vi "数据查询_仪器数据.vi"() -> ()   [LabVIEW 2016]
uses:
  <vilib>/Utility/miscctls.llb/LVRowAndColumnUnsignedTypeDef.ctl
  <vilib>/Utility/miscctls.llb/LVPointTypeDef.ctl
  <userlib>/_OpenG.lib/array/array.llb/Sort 2D Array (String)__ogtk.vi
panel:
  in  "序列号":string
  out "总共行数":i32
  in  "显示行数":i32=15
  in  "下拉列表":string(xcontrol)
  in  "导出":bool
  out "分钟小时":string(combo)="实时数据"
  out "工作类型":string(combo)="全部数据"
  in  "查询":bool
  in  "结束日期":string="2050/01/01"
  in  "起始日期":string="2010/01/01"
  out "数据表":string[][](table)
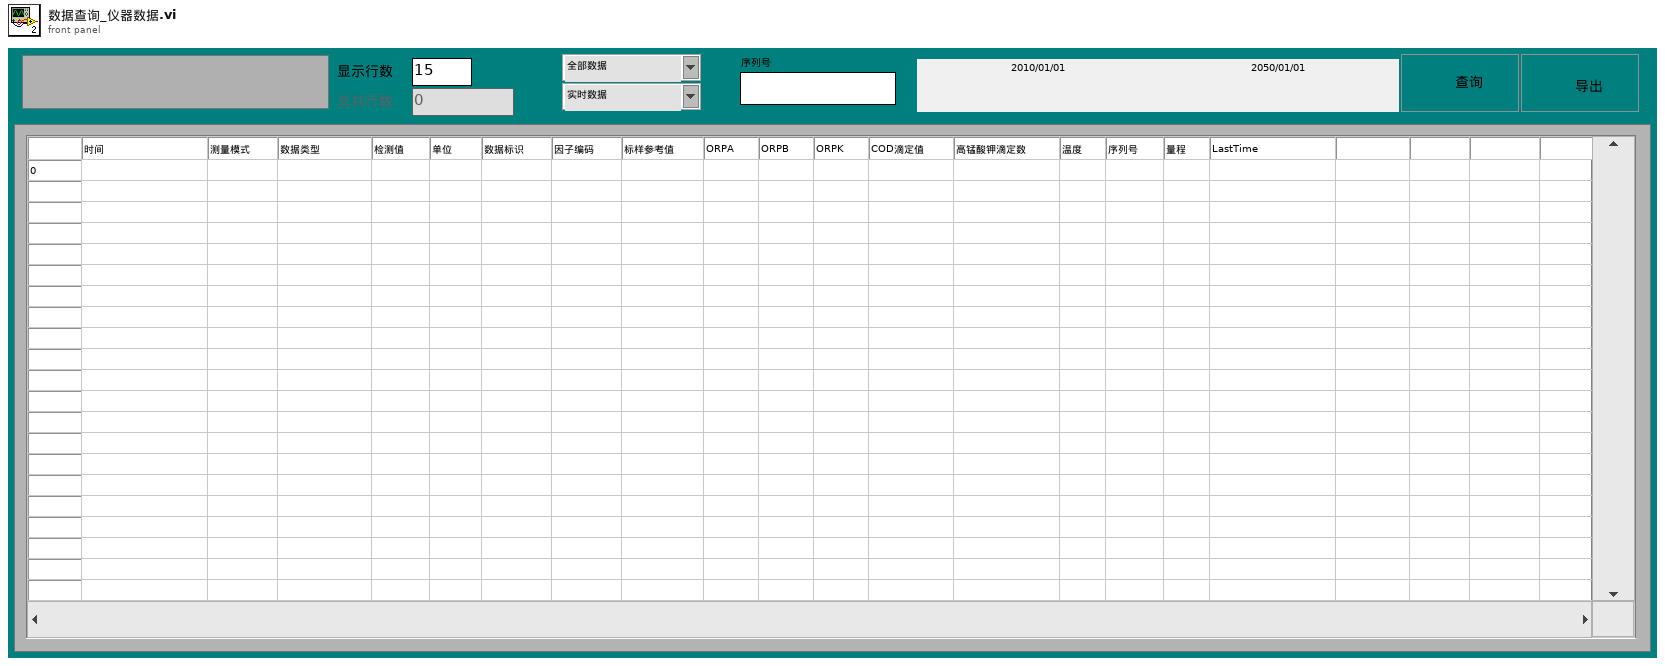
[diagram p1: front panel]
types:
  T1 = enum8{"Enabled", "Disabled", "Disabled and Grayed Out"}
  T2 = typedef "LVRowAndColumnUnsignedTypeDef.ctl" = cluster{"Row":u32, "Column":u32}
  T3 = typedef "LVPointTypeDef.ctl" = cluster{"Horizontal":i16, "Vertical":i16}
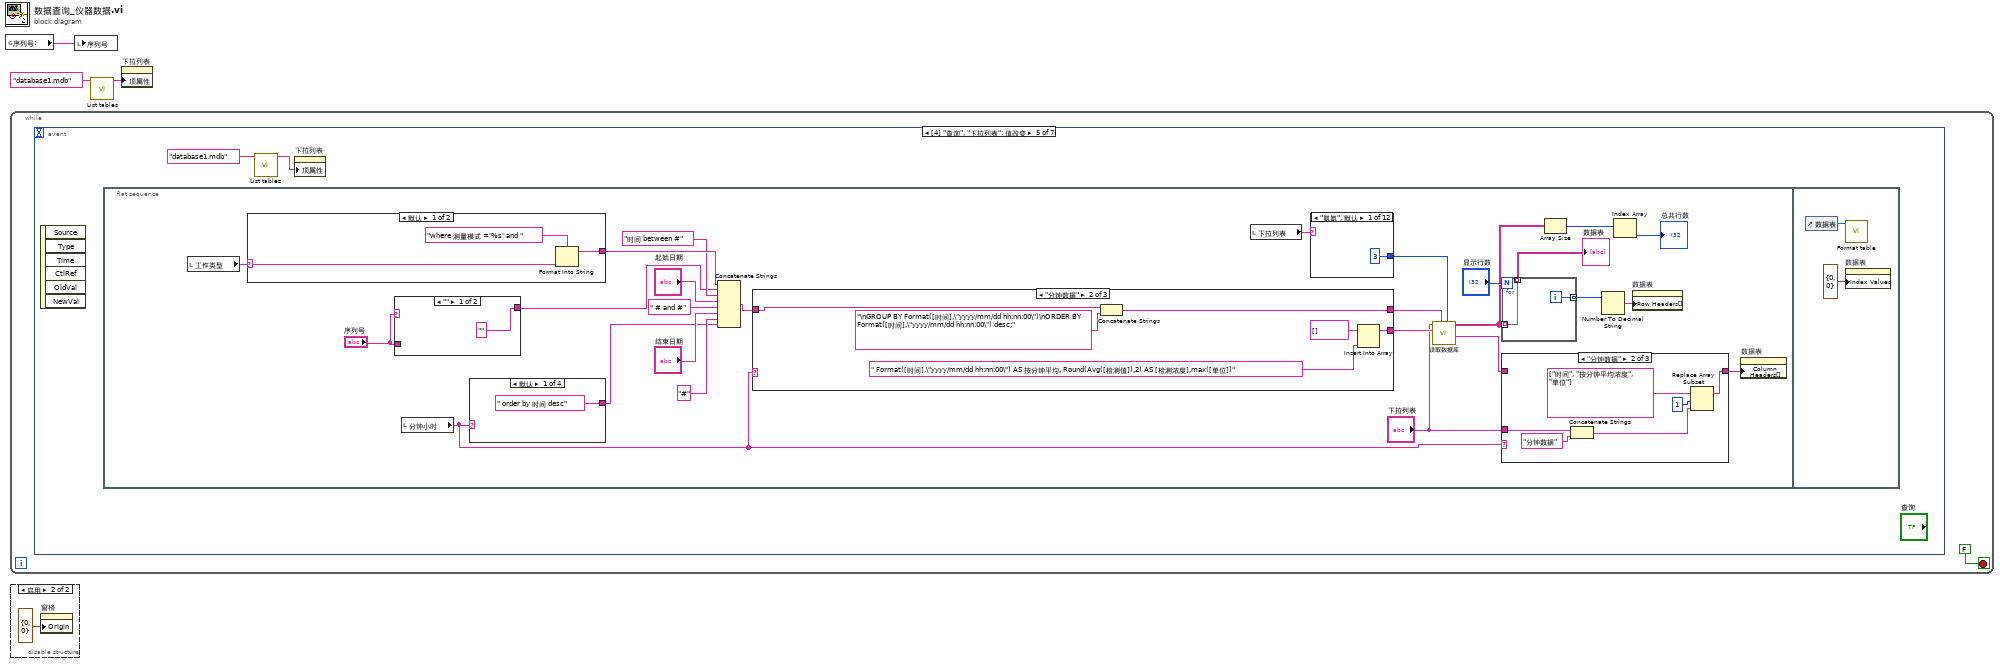
[diagram p0: block diagram]
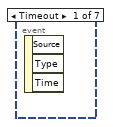
[diagram p2: hidden frame]
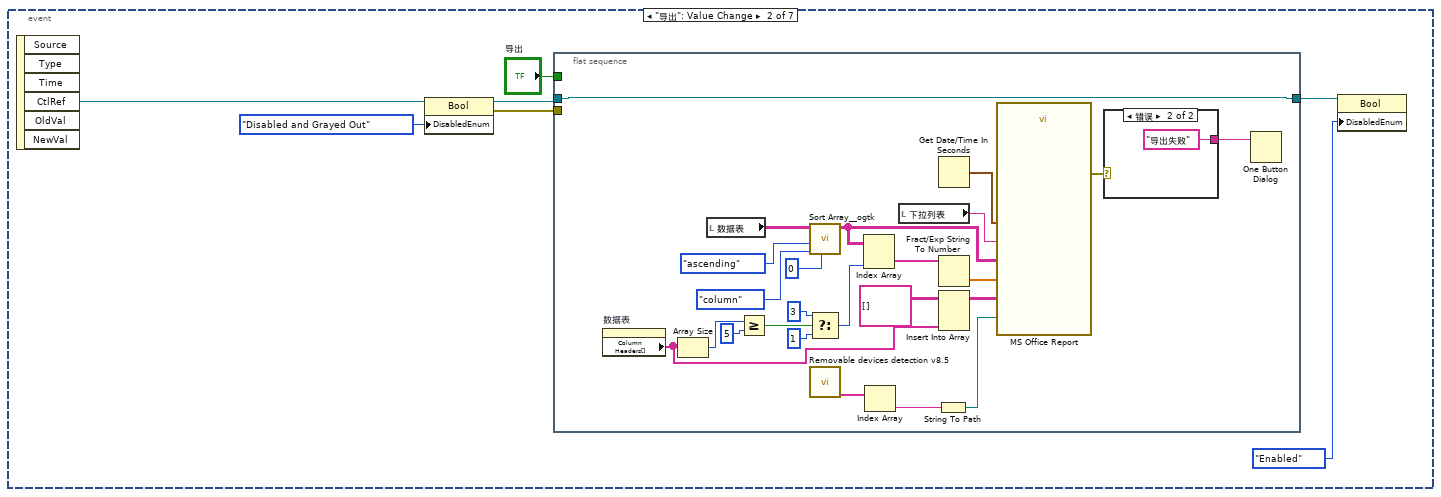
[diagram p3: hidden frame]
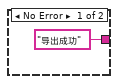
[diagram p4: hidden frame]
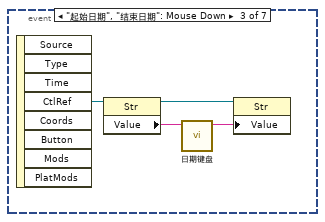
[diagram p5: hidden frame]
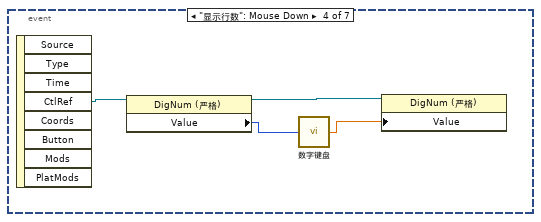
[diagram p6: hidden frame]
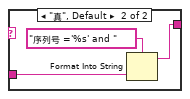
[diagram p7: hidden frame]
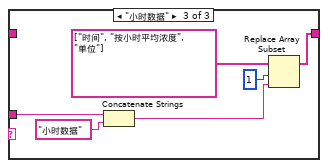
[diagram p9: hidden frame]
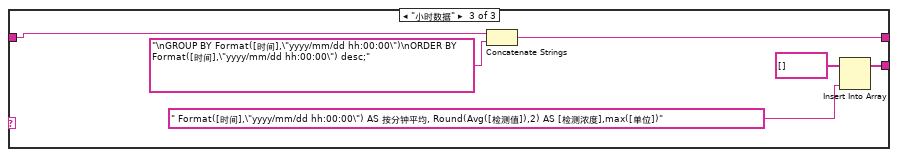
[diagram p14: hidden frame]
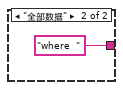
[diagram p15: hidden frame]
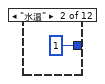
[diagram p16: hidden frame]
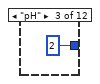
[diagram p17: hidden frame]
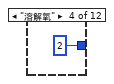
[diagram p18: hidden frame]
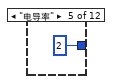
[diagram p19: hidden frame]
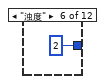
[diagram p20: hidden frame]
diagram:
  n1 = global read "COD内部交互全局.vi" "序列号:"() -> (w1:string)
  n2 = while {
    stop <- FALSE stop-if-true
    n3 = event shown="[4] \"查询\", \"下拉列表\": 值改变" {
      selector: _ -> [_ _ _ _ _ _ _]
      dyn-events: _ -> [_ _ _ _ _ _ _]
      timeout: _ -> [_ _ _ _ _ _ _]
      event Timeout {
        n4 = event-data() -> ()  [unwired: 1 in, 3 out]
      }
      event "导出": Value Change {
        n5 = event-data() -> ("CtlRef"=w5:refnum<vi>)  [unwired: 1 in, 5 out]
        n6 = property class="Bool"(reference=w5, "DisabledEnum"=T1."Disabled and Grayed Out" ("禁用")) -> (reference out=w9:refnum<vi>, error out=w10:errorcluster)  [unwired: 1 in]
        n7 = flat-sequence {
          tunnel: w10 -> [_]
          tunnel: [w26] -> w8
          tunnel: w9 -> [w26]
          tunnel: "导出" -> [_]
          frame #0 {
            n8 = property on="数据表" class="Tbl (严格)"() -> ("Column Headers[]"=w13:string[])  [unwired: 2 in, 2 out]
            n9 = Array Size(array=w13) -> (size(s)=w20:i32)
            n10 = local read "数据表"() -> (w34:string[][])
            n11 = Greater Or Equal?(x=w20, y=5) -> (x >= y?=w18:bool)
            n12 = call-poly <userlib>:"Sort Array__ogtk.vi"("Column/Row to Sort By"=u32 0, "Sort By in"=enum16{"row", "column"}."column", "Order"=enum16{"ascending", "descending"}."ascending", "Array in"=w34) -> ("Sorted Array out"=w33:string[][])  [unwired: 4 in, 3 out]
            n13 = Select(t=3 ("禁用的索引 (列)"), s=w18, f=1) -> (s? t:f=w16:i32)
            n14 = call "Removable devices detection v8.5.vi"() -> ("Removable"=w23:string[])  [unwired: 4 out]
            n15 = Index Array(array=w33, index (col)=w16) -> (element=w29:string[])  [unwired: 1 in]
            n16 = Index Array(array=w23) -> (element=w22:string)  [unwired: 1 in]
            n17 = local read "下拉列表"() -> (w27:string)
            n18 = String To Path(string=w22) -> (path=w21:path)
            n19 = Get Date/Time In Seconds() -> (seconds since 1Jan1904=w35:timestamp)
            n20 = Fract/Exp String To Number(string=w29) -> (number=w28:dbl[])  [unwired: 3 in, 1 out]
            n21 = Insert Into Array(array=string[][] [], new element=w13) -> (w12:string[][])  [unwired: 2 in]
            n22 = call "MS Office Report"("Path to Save Report"=w21, "导出日期"=w35, "监测参数"=w27, "数据输入"=w33, "图表输入"=w28, "字段定义"=w12) -> ("error out"=w25:errorcluster)  [unwired: 20 in, 1 out]
            n23 = case shown="错误" w25 {
              tunnel: ["导出成功" ("消息") "导出失败" ("消息")] -> w24
              frame No Error {
              }
              frame Error {
              }
            }
            n24 = One Button Dialog(message=w24) -> ()  [unwired: 1 in, 1 out]
          }
        }
        n25 = property class="Bool"(reference=w8, "DisabledEnum"=T1."Enabled" ("禁用")) -> ()  [unwired: 1 in, 2 out]
      }
      event "起始日期", "结束日期": Mouse Down {
        n26 = event-data() -> ("CtlRef"=w41:refnum<vi>)  [unwired: 1 in, 7 out]
        n27 = property class="Str"(reference=w41) -> (reference out=w39:refnum<vi>, "Value"=w40:string)  [unwired: 1 in, 1 out]
        n28 = call "日期键盘.vi"("原值"=w40) -> ("x+y"=w38:string)  [unwired: 10 in]
        n29 = property class="Str"(reference=w39, "Value"=w38) -> ()  [unwired: 1 in, 2 out]
      }
      event "显示行数": Mouse Down {
        n30 = event-data() -> ("CtlRef"=w45:refnum<vi>)  [unwired: 1 in, 7 out]
        n31 = property class="DigNum (严格)"(reference=w45) -> (reference out=w44:refnum<vi>, "Value"=w43:i32)  [unwired: 1 in, 1 out]
        n32 = call "数字键盘.vi"("OldNumber"=w43) -> ("NewNumber"=w42:sgl)
        n33 = property class="DigNum (严格)"(reference=w44, "Value"=w42) -> ()  [unwired: 1 in, 2 out]
      }
      event "查询", "下拉列表": Value Change {
        n34 = event-data() -> ()  [unwired: 1 in, 6 out]
        n35 = flat-sequence {
          frame #0 {
            n36 = local read "工作类型"() -> (w65:string)
            n37 = case shown="默认" w65 {
              selector: w65 -> [w107 _]
              tunnel: [w105 "where  " ("condition")] -> w50
              frame Default {
                n38 = Format Into String(format string="where 测量模式 ='%s' and " ("condition"), w107) -> (resulting string=w105:string)  [unwired: 2 in, 1 out]
              }
              frame "全部数据" {
              }
            }
            n39 = case shown="\"\"" "序列号" {
              tunnel: "序列号" -> [_ w76]
              tunnel: ["" ("condition") w75] -> w48
              frame "" {
              }
              frame "真", Default {
                n40 = Format Into String(format string="序列号 ='%s' and " ("condition"), w76) -> (resulting string=w75:string)  [unwired: 2 in, 1 out]
              }
            }
            n41 = local read "分钟小时"() -> (w60:string)
            n42 = case shown="默认" w60 {
              tunnel: [" order by 时间 desc" ("字符串") _ _ _] -> w64
              frame Default {
              }
              frame "分钟数据" {
              }
              frame "小时数据" {
              }
              frame "真" {
              }
            }
            n43 = Concatenate Strings(w50, w48, "时间 between #" ("condition"), "起始日期", " # and #" ("condition"), "结束日期", "#" ("condition"), w64) -> (w63:string)
            n44 = case shown="\"分钟数据\"" w60 {
              tunnel: [_ w97 w99] -> w61
              tunnel: w63 -> [w92 w95 w101]
              tunnel: [w92 w94 w100] -> w62
              frame Default {
              }
              frame "分钟数据" {
                n45 = Concatenate Strings(w95, "\nGROUP BY Format([时间],\"yyyy/mm/dd hh:nn:00\")\nORDER BY Format([时间],\"yyyy/mm/dd hh:nn:00\") desc;" ("字符串")) -> (w94:string)
                n46 = Insert Into Array(array=string[] [] ("显示项"), new element=" Format([时间],\"yyyy/mm/dd hh:nn:00\") AS 按分钟平均, Round(Avg([检测值]),2) AS [检测浓度],max([单位])" ("新元素/子数组")) -> (w97:string[])  [unwired: 1 in]
              }
              frame "小时数据" {
                n47 = Concatenate Strings(w101, "\nGROUP BY Format([时间],\"yyyy/mm/dd hh:00:00\")\nORDER BY Format([时间],\"yyyy/mm/dd hh:00:00\") desc;" ("字符串")) -> (w100:string)
                n48 = Insert Into Array(array=string[] [] ("显示项"), new element=" Format([时间],\"yyyy/mm/dd hh:00:00\") AS 按分钟平均, Round(Avg([检测值]),2) AS [检测浓度],max([单位])" ("新元素/子数组")) -> (w99:string[])  [unwired: 1 in]
              }
            }
            n49 = local read "下拉列表"() -> (w67:string)
            n50 = case shown="\"氨氮\", 默认" w67 {
              tunnel: [i16 3 ("精度(6)") i16 1 ("精度(6)") i16 2 ("精度(6)") i16 2 ("精度(6)") i16 2 ("精度(6)") i16 2 ("精度(6)") i16 2 ("精度(6)") i16 2 ("精度(6)") i16 3 ("精度(6)") i16 2 ("精度(6)") i16 2 ("精度(6)") i16 2 ("精度(6)")] -> w66
              frame "氨氮", Default {
              }
              frame "水温" {
              }
              frame "pH" {
              }
              frame "溶解氧" {
              }
              frame "电导率" {
              }
              frame "浊度" {
              }
              frame "藻密度" {
              }
              frame "叶绿素a" {
              }
              frame "总磷" {
              }
              frame "总氮" {
              }
              frame "CodCr" {
              }
              frame "CodMn" {
              }
            }
            n51 = call "读取数据库.vi"("精度(6)"=w66, "condition"=w62, "显示项"=w61, "组合框"="下拉列表") -> ("columns"=w59:string[], "表格"=w52:string[][])  [unwired: 4 in, 2 out]
            n52 = for {
              N: "显示行数" -> [_]
              tunnel: w52 -> [w121] mode=indexing
              tunnel: [w122] -> w69 mode=indexing
              tunnel: [w121] -> w55 mode=indexing
              i -> [w122]
            }
            "数据表" <- w55
            n53 = case shown="\"分钟数据\"" w60 {
              tunnel: w59 -> [w78 _ _]
              tunnel: [w78 w82 w86] -> w58
              tunnel: "下拉列表" -> [_ w81 w87]
              frame Default {
              }
              frame "分钟数据" {
                n54 = Concatenate Strings(w81, "分钟数据" ("字符串")) -> (w79:string)
                n55 = Replace Array Subset(array=string[] ["时间", "按分钟平均浓度", "单位"] ("columns"), new element=w79, index=1 ("索引")) -> (w82:string[])
              }
              frame "小时数据" {
                n56 = Concatenate Strings(w87, "小时数据" ("字符串")) -> (w88:string)
                n57 = Replace Array Subset(array=string[] ["时间", "按小时平均浓度", "单位"] ("columns"), new element=w88, index=1 ("索引")) -> (w86:string[])
              }
            }
            n58 = Array Size(array=w52) -> (size(s)=w54:i32[])
            n59 = Number To Decimal String(number=w69) -> (decimal integer string=w68:string[])  [unwired: 1 in]
            n60 = Index Array(array=w54) -> (element=→"总共行数":i32)  [unwired: 1 in]
            n61 = property on="数据表" class="Tbl (严格)"("Row Headers[]"=w68) -> ()  [unwired: 2 in, 2 out]
            n62 = property on="数据表" class="Tbl (严格)"("Column Headers[]"=w58) -> ()  [unwired: 2 in, 2 out]
          }
          frame #1 {
            n63 = control-ref of="数据表"() -> (w123:refnum<vi>)
            n64 = call "Format table.vi"("Table输入"=w123) -> ()  [unwired: 11 in]
            n65 = property on="数据表" class="Tbl (严格)"("Index Values"=T2 {"Row"=0, "Column"=0} ("索引值")) -> ()  [unwired: 2 in, 2 out]
          }
        }
        n66 = call "List tables.vi"("database"="database1.mdb") -> ("tables"=w46:string[])  [unwired: 9 in, 1 out]
        n67 = property on="下拉列表" class="下拉列表 (严格)"("项属性"=w46) -> ()  [unwired: 2 in, 2 out]
      }
      event "工作类型", "分钟小时": Mouse Down {
        n68 = event-data() -> ()  [unwired: 1 in, 8 out]
        n69 = call "数据查询筛选.vi"() -> ("分钟小时"=→"分钟小时":string, "工作类型"=→"工作类型":string)  [unwired: 10 in]
      }
      event "序列号": Mouse Down {
        n70 = event-data() -> ("CtlRef"=w127:refnum<vi>)  [unwired: 1 in, 7 out]
        n71 = property class="Str"(reference=w127) -> (reference out=w131:refnum<vi>, "Value"=w132:string)  [unwired: 1 in, 1 out]
        n72 = Two Button Dialog(message="查询所有序列号？" ("消息")) -> (T button?=w128:bool)  [unwired: 2 in]
        n73 = case shown="假" w128 {
          tunnel: w132 -> [w134 _]
          tunnel: [w133 "" ("x+y")] -> w130
          frame False {
            n74 = call "字符键盘.vi"("原值"=w134) -> ("x+y"=w133:string)  [unwired: 10 in]
          }
          frame True {
          }
        }
        n75 = property class="Str"(reference=w131, "Val(Sgnl)"=w130) -> ()  [unwired: 1 in, 2 out]
      }
    }
  }
  n76 = disable-structure shown="启用" {
    frame Disabled {
    }
    frame Enabled {
      n77 = property on="窗格" class="Pane"("Origin"=T3 {"Horizontal"=0, "Vertical"=0} ("原点")) -> ()  [unwired: 2 in, 2 out]
    }
  }
  n78 = local write "序列号"(w1) -> ()
  n79 = call "List tables.vi"("database"="database1.mdb") -> ("tables"=w2:string[])  [unwired: 9 in, 1 out]
  n80 = property on="下拉列表" class="下拉列表 (严格)"("项属性"=w2) -> ()  [unwired: 2 in, 2 out]
